vi "say_hello.vi"(8 "error in (no error)":errorcluster, 11 "WebSocket in":refnum<class "WebSocket.lvclass">) -> (0 "error out":errorcluster, 3 "WebSocket out":refnum<class "WebSocket.lvclass">)   [LabVIEW 2018]
uses:
  <vilib>/MediaMongrels Ltd/WebSockets/WebSockets/WebSocket/WebSocket.lvclass
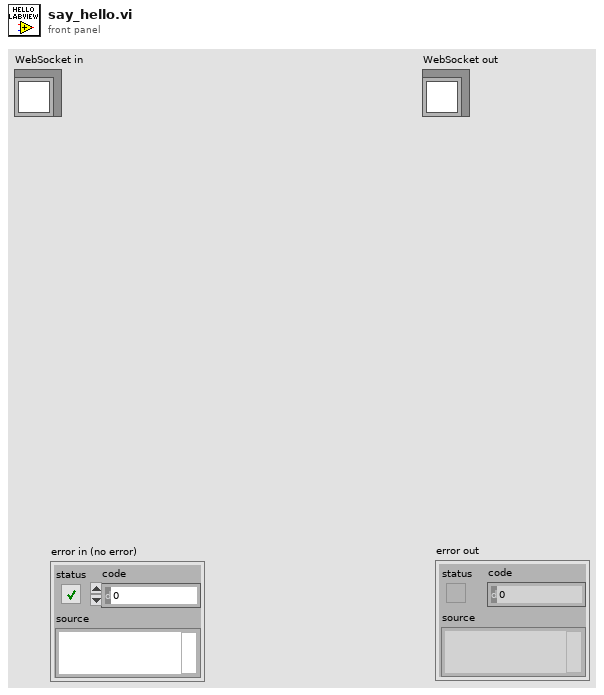
[diagram p1: front panel]
types:
  T1 = cluster{"cmd":string, "data":string, "dtype":string}
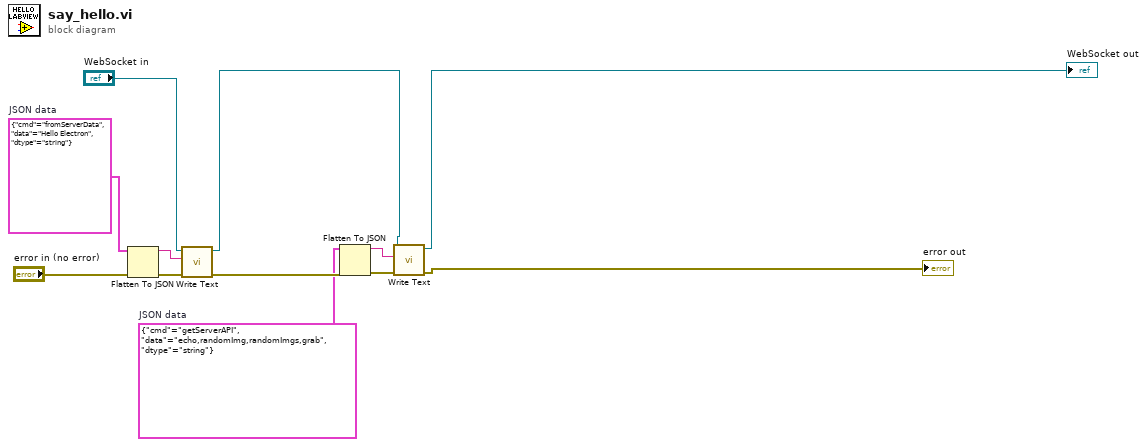
[diagram p0: block diagram]
diagram:
  w1 = T1 {"cmd"="getServerAPI", "data"="echo,randomImg,randomImgs,grab", "dtype"="string"}  # JSON data
  w10 = T1 {"cmd"="fromServerData", "data"="Hello Electron", "dtype"="string"}  # JSON data
  n1 = Flatten To JSON(anything=w10, error in (no error)="error in (no error)") -> (JSON string=w11:string, 11:w12:errorcluster)  [unwired: 1 in]
  n2 = call-dynamic "Write Text.vi"("error in (no error)"=w12, "String Data"=w11, "WebSocket in"="WebSocket in") -> ("error out"=w5:errorcluster, "WebSocket out"=w3:refnum<class "WebSocket.lvclass">)  [unwired: 7 in]
  n3 = Flatten To JSON(anything=w1, error in (no error)=w5) -> (JSON string=w6:string, 11:w7:errorcluster)  [unwired: 1 in]
  n4 = call-dynamic "Write Text.vi"("error in (no error)"=w7, "String Data"=w6, "WebSocket in"=w3) -> ("error out"=→"error out":errorcluster, "WebSocket out"=→"WebSocket out":refnum<class "WebSocket.lvclass">)  [unwired: 7 in]
